vi "test Multi FPGA Feature Toggle No Bitfile.vi"(8 "error in (no error)":errorcluster, 11 "TestCase in":refnum<class "Mutation Test Case.lvclass">) -> (0 "error out":errorcluster, 3 "TestCase out":refnum<class "Mutation Test Case.lvclass">)   [LabVIEW 2015, in "Mutation Test Case.lvclass"]
uses:
  Mutation Test Case.lvclass
  Shared/Properties.vi
  <vilib>/NI Veristand/Custom Device API/Get Item Property (String).vi
  <vilib>/NI Veristand/Custom Device API/Get Item Property (Boolean).vi
  <vilib>/addons/_JKI Toolkits/VI Tester/TestCase.llb/TestCase.lvclass
  System Explorer/Engine Simulation Toolkit System Explorer.lvlib
  <vilib>/NI VeriStand/Custom Device API/Custom Device API.lvlib
  Shared/Engine Simulation Toolkit Shared.lvlib
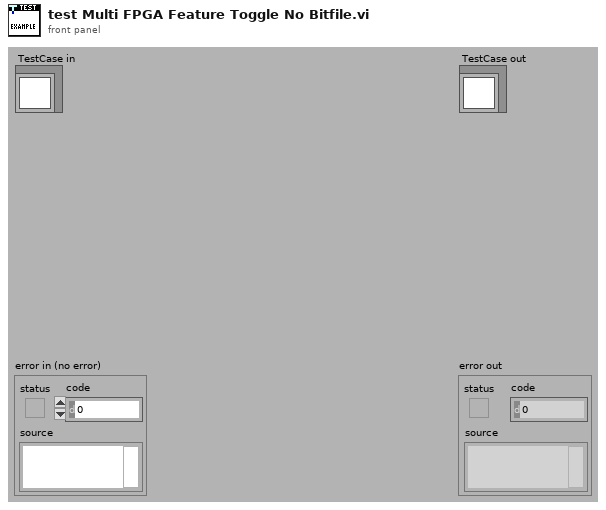
[diagram p1: front panel]
types:
  T1 = typedef "Custom Device API.lvlib/Custom Device Item Ref.ctl" = u64
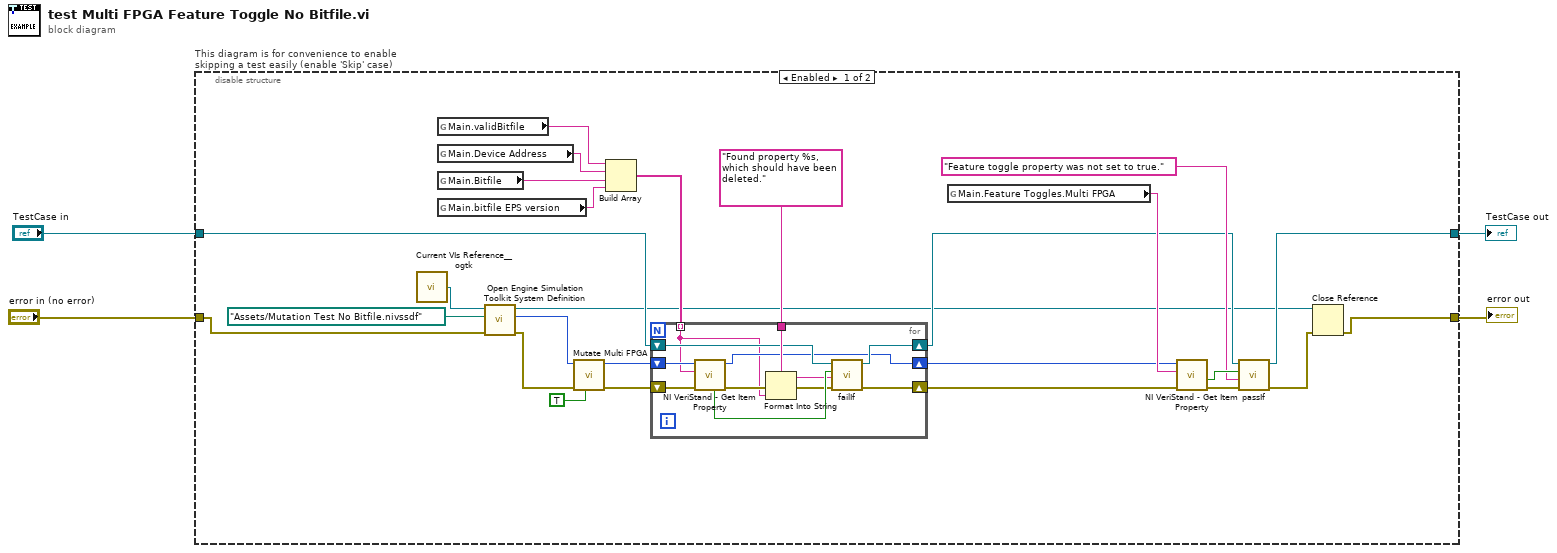
[diagram p0: block diagram]
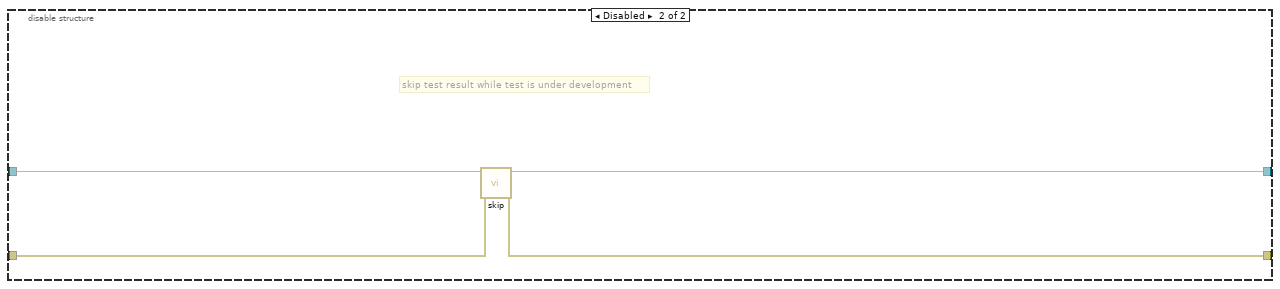
[diagram p2: hidden frame]
diagram:
  n1 = disable-structure "This diagram is for convenience to enable skipping a test easily (enable 'Skip' case)" shown="Enabled" {
    disable-tunnel: "TestCase in" -> [w24 w46]
    disable-tunnel: [w13 w44] -> w1
    disable-tunnel: [w6 w45] -> w3
    disable-tunnel: "error in (no error)" -> [w28 w43]
    frame Enabled {
      n2 = call <userlib>:"Current VIs Reference__ogtk.vi"() -> ("Current VI's reference"=w30:refnum<vi>)  [unwired: 5 in]
      n3 = global read "Properties.vi" "Main.validBitfile"() -> (w21:string)
      n4 = global read "Properties.vi" "Main.Device Address"() -> (w22:string)
      n5 = global read "Properties.vi" "Main.Bitfile"() -> (w20:string)
      n6 = global read "Properties.vi" "Main.bitfile EPS version"() -> (w19:string)
      n7 = call "Open Engine Simulation Toolkit System Definition.vi"("error in (no error)"=w28, "System Definition Path"=path "Assets/Mutation Test No Bitfile.nivssdf" ("Absolute or Relative Path"), "Current VI in"=w30) -> ("error out"=w8:errorcluster, "Engine Simulation Toolkit NodeID"=w27:u64, "SystemDefinition"=w5:refnum<k24>)  [unwired: 6 in]
      n8 = call "Mutate Multi FPGA.vi"("Force (F)"=TRUE, "error in (no error)"=w8, "Device Ref in"=w27) -> ("error out"=w25:errorcluster, "Device Ref out"=w26:T1)  [unwired: 7 in]
      n9 = Build Array(w21, w22, w20, w19) -> (w18:string[])
      n10 = for {
        shift-right: [w38] -> w15
        shift-left: w25 -> [w41]
        shift-right: [w39] -> w9
        shift-left: w24 -> [w36]
        tunnel: w18 -> [w31] mode=indexing
        tunnel: "Found property %s, which should have been deleted." ("format string") -> [w37]
        shift-right: [w32] -> w14
        shift-left: w26 -> [w42]
        n11 = call-poly <vilib>:"NI VeriStand - Get Item Property.vi"("error in (no error)"=w41, "Property Name"=w31, "Item Ref in"=w42) -> ("error out"=w35:errorcluster, "Item Ref out"=w32:T1, "Found?"=w40:bool)  [unwired: 5 in, 1 out]
        n12 = Format Into String(format string=w37, error in=w35, w31) -> (resulting string=w33:string, error out=w34:errorcluster)  [unwired: 1 in]
        n13 = call-dynamic "failIf.vi"("error in (no error)"=w34, "message (\"\")"=w33, "fail"=w40, "TestCase in"=w36) -> ("error out"=w38:errorcluster, "TestCase out"=w39:refnum<class "Mutation Test Case.lvclass">)  [unwired: 6 in]
      }
      n14 = global read "Properties.vi" "Main.Feature Toggles.Multi FPGA"() -> (w16:string)
      n15 = call-poly <vilib>:"NI VeriStand - Get Item Property.vi"("error in (no error)"=w15, "Property Name"=w16, "Item Ref in"=w14) -> ("error out"=w12:errorcluster, "Value"=w11:bool)  [unwired: 5 in, 2 out]
      n16 = call-dynamic "passIf.vi"("error in (no error)"=w12, "message (\"\")"="Feature toggle property was not set to true." ("message (\"\")"), "pass"=w11, "TestCase in"=w9) -> ("error out"=w7:errorcluster, "TestCase out"=w13:refnum<class "Mutation Test Case.lvclass">)  [unwired: 6 in]
      n17 = Close Reference(reference=w5, error in (no error)=w7) -> (error out=w6:errorcluster)
    }
    frame Disabled {
      # "skip test result while test is under development"
      n18 = call <vilib>:"skip.vi"("error in (no error)"=w43, "TestCase in"=w46) -> ("error out"=w45:errorcluster, "TestCase out"=w44:refnum<class "Mutation Test Case.lvclass">)  [unwired: 8 in]
    }
  }
  "error out" <- w3
  "TestCase out" <- w1
